vi "Read (Multiple Waveforms).vi"(7 "Segment Index (0)":i32 format="%.0g", 8 "error in (no error)":errorcluster, 9 "Maximum Time (10000ms)":u32, 10 "Channels":i32[](array[ring]) items=["Channel 1", "Channel 2", "Channel 3", "Channel 4", "Function 1", "Function 2", "Function 3", "Function 4", "Memory 1", "Memory 2", "Memory 3", "Memory 4"], 11 "VISA resource name":refnum<visa-resource-name>) -> (0 "error out":errorcluster, 2 "Waveform Data":waveform(dbl)[](graph), 3 "VISA resource name out":refnum<visa-resource-name>)   [LabVIEW 2009, in "Agilent 8000 Series.lvlib"]
doc: "Initiates an acquisition on all channels that you enabled with the Configure Channel VI. The VI waits for the acquisition to complete and returns the waveform for the <B>Source Channel</B> you specified. If the oscilloscope did not complete the acquisition within the time period you specify with the <B>Timeout</B> control, the VI returns a timeout error. A common cause for a timeout error is the acquisition was not triggered. For example, the trigger level is out of range of the waveform. If the sampling mode is set to segment, you can set the <B>Segment Index</B>.\n\n<B>Note:</B> If your instrument does not support auto compensation for probe attenuation, you may need to adjust the scaling of the waveform data accordingly. This is handled automatically in the Configure Channel VI or can be done manually by multiplying the waveform data by the probe attenuation."
uses:
  Agilent 8000 Series.lvlib
  Low Level/Fetch (Waveform).vi
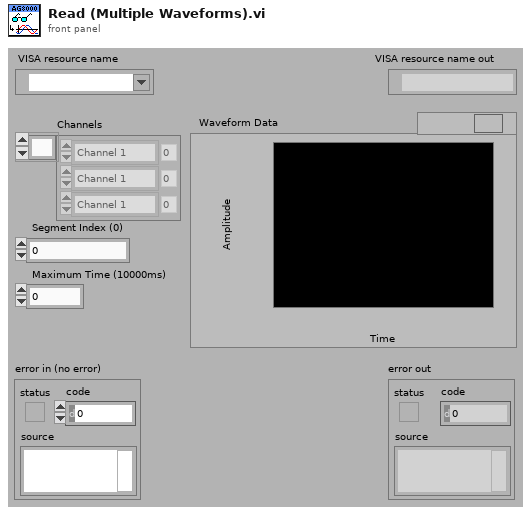
[diagram p1: front panel]
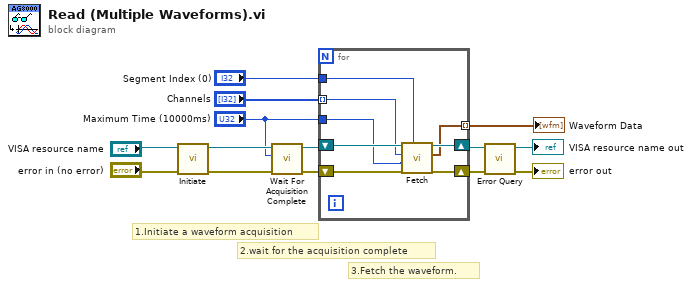
[diagram p0: block diagram]
diagram:
  # "3.Fetch the waveform."
  # "2.wait for the acquisition complete"
  # "1.Initiate a waveform acquisition"
  n1 = call "Initiate.vi"("error in (no error)"="error in (no error)", "VISA resource name"="VISA resource name") -> ("error out"=w5:errorcluster, "VISA resource name out"=w6:refnum<visa-resource-name>)  [unwired: 8 in]
  n2 = call "Wait For Acquisition Complete.vi"("error in (no error)"=w5, "Maximum Time (10000ms)"="Maximum Time (10000ms)", "VISA resource name"=w6) -> ("error out"=w4:errorcluster, "VISA resource name out"=w3:refnum<visa-resource-name>)  [unwired: 7 in]
  n3 = for {
    shift-right: [w20] -> w11
    shift-left: w4 -> [w19]
    tunnel: [w17] -> w8 mode=indexing
    tunnel: "Maximum Time (10000ms)" -> [w18]
    shift-right: [w21] -> w12
    shift-left: w3 -> [w22]
    tunnel: "Segment Index (0)" -> [w16]
    tunnel: "Channels" -> [w15] mode=indexing
    n4 = call-poly "Fetch.vi"("Segment Index (0)"=w16, "error in (no error)"=w19, "Maximum Time (10000ms)"=w18, "Channel (1: Channel 1)"=w15, "VISA resource name"=w22) -> ("error out"=w20:errorcluster, "Waveform Data"=w17:waveform(dbl), "VISA resource name out"=w21:refnum<visa-resource-name>)  [unwired: 4 in]
  }
  "Waveform Data" <- w8
  n5 = call "Error Query.vi"("error in (no error)"=w11, "VISA resource name"=w12) -> ("error out"=→"error out":errorcluster, "VISA resource name out"=→"VISA resource name out":refnum<visa-resource-name>)  [unwired: 6 in, 2 out]
